vi "Untitled 2.vi"() -> ()   [LabVIEW 2022 SP3]
panel:
  out "standard output":string
  out "standard error":string
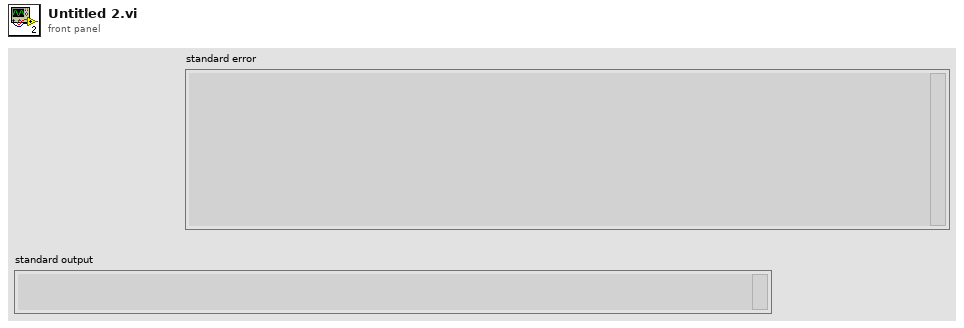
[diagram p1: front panel]
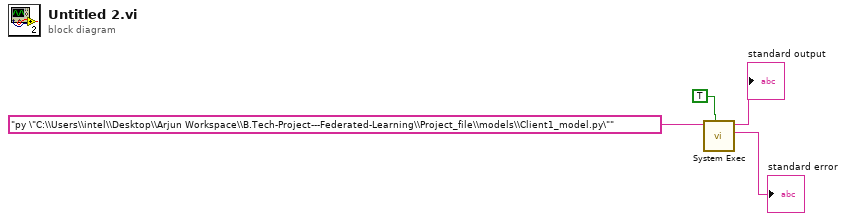
[diagram p0: block diagram]
diagram:
  n1 = call <vilib>:"System Exec.vi"("wait until completion? (T)"=TRUE, "command line"="py \"C:\\Users\\intel\\Desktop\\Arjun Workspace\\B.Tech-Project---Federated-Learning\\Project_file\\models\\Client1_model.py\"") -> ("standard error"=→"standard error":string, "standard output"=→"standard output":string)  [unwired: 6 in, 2 out]
